vi "PSTR-Get Raw Metrics.vi"(0 "PSTH":dbl[](array[numeric]), 7 "dt (ms)":dbl, 9 "delay (ms)":dbl, 11 "durat (ms)":dbl) -> (8 "metrics":T1)   [LabVIEW 2020]
uses:
  <vilib>/Analysis/baseanly.llb/Mean (DBL).vi
  <vilib>/Analysis/NI_AALBase.lvlib
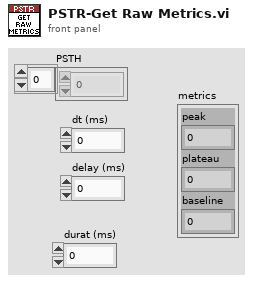
[diagram p1: front panel]
types:
  T1 = cluster{"peak":dbl, "plateau":dbl, "baseline":dbl}
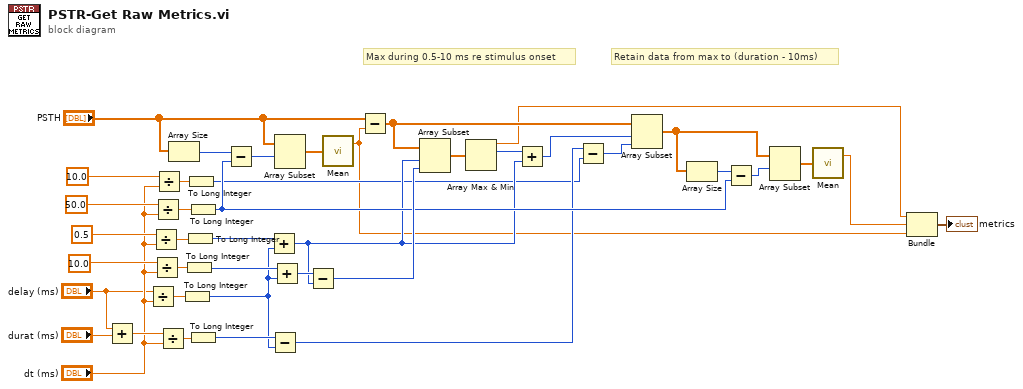
[diagram p0: block diagram]
diagram:
  # "Retain data from max to (duration - 10ms)"
  # "Max during 0.5-10 ms re stimulus onset"
  n1 = Add(x="delay (ms)", y="durat (ms)") -> (x+y=w39:dbl)
  n2 = Divide(x="delay (ms)", y="dt (ms)") -> (x/y=w41:dbl)
  n3 = Divide(x=0.5, y="dt (ms)") -> (x/y=w35:dbl)
  n4 = Divide(x=10.0, y="dt (ms)") -> (x/y=w34:dbl)
  n5 = Divide(x=50.0, y="dt (ms)") -> (x/y=w25:dbl)
  n6 = Divide(x=10.0, y="dt (ms)") -> (x/y=w9:dbl)
  n7 = Divide(x=w39, y="dt (ms)") -> (x/y=w38:dbl)
  n8 = Array Size(array="PSTH") -> (size(s)=w23:i32)
  n9 = To Long Integer(number=w41) -> (32bit integer=w27:i32)
  n10 = To Long Integer(number=w34) -> (32bit integer=w33:i32)
  n11 = To Long Integer(number=w35) -> (32bit integer=w12:i32)
  n12 = To Long Integer(number=w9) -> (32bit integer=w8:i32)
  n13 = To Long Integer(number=w25) -> (32bit integer=w17:i32)
  n14 = To Long Integer(number=w38) -> (32bit integer=w28:i32)
  n15 = Subtract(x=w23, y=w17) -> (x-y=w20:i32)
  n16 = Add(x=w12, y=w27) -> (x+y=w15:i32)
  n17 = Subtract(x=w28, y=w27) -> (x-y=w13:i32)
  n18 = Add(x=w33, y=w27) -> (x+y=w29:i32)
  n19 = Array Subset(array="PSTH", index=w20) -> (w22:dbl[])  [unwired: 1 in]
  n20 = Subtract(x=w29, y=w15) -> (x-y=w32:i32)
  n21 = call-poly <vilib>:"Mean.vi"("X"=w22) -> ("mean"=w2:dbl)  [unwired: 1 out]
  n22 = Subtract(x="PSTH", y=w2) -> (x-y=w21:dbl[])
  n23 = Array Subset(array=w21, index=w15, length=w32) -> (w31:dbl[])
  n24 = Array Max & Min(array=w31) -> (max value=w4:dbl, max index (indices)=w30:i32)  [unwired: 2 out]
  n25 = Add(x=w30, y=w15) -> (x+y=w14:i32)
  n26 = Subtract(x=w13, y=w8) -> (x-y=w7:i32)
  n27 = Array Subset(array=w21, index=w14, length=w7) -> (w16:dbl[])
  n28 = Array Size(array=w16) -> (size(s)=w19:i32)
  n29 = Subtract(x=w19, y=w17) -> (x-y=w18:i32)
  n30 = Array Subset(array=w16, index=w18) -> (w6:dbl[])  [unwired: 1 in]
  n31 = call-poly <vilib>:"Mean.vi"("X"=w6) -> ("mean"=w3:dbl)  [unwired: 1 out]
  n32 = Bundle(w4, "mean"=w3, "mean"=w2) -> (→"metrics":cluster{dbl, "mean":dbl, "mean":dbl})  [unwired: 1 in]
